vi "from string.vi"(8 "error in":errorcluster, 9 "data":string, 10 "version":string, 11 "Special Test configuration":refnum<class "Special Test configuration.lvclass">) -> (0 "error out":errorcluster, 3 "Special Test configuration out":refnum<class "Special Test configuration.lvclass">)   [LabVIEW 2025, in "Special Test.lvlib" / "Special Test configuration.lvclass"]
doc: "Provides an interface for loading a module configuration from a file or other serialized data source. It is recommended that all children of this class store data in two sets--data required for its own initialization, and any data required for parent initialization--and that each implementation uses the <b>Call Parent Method</b> primitive to de-serialize parent information.Copyright 2017 National Instruments Corporation\n\nLicensed under the Apache License, Version 2.0 (the \"License\"); you may not use this file except in compliance with the License. You may obtain a copy of the License at http://www.apache.org/licenses/LICENSE-2.0\nUnless required by applicable law or agreed to in writing, software distributed under the License is distributed on an \"AS IS\" BASIS, WITHOUT WARRANTIES OR CONDITIONS OF ANY KIND, either express or implied. See the License for the specific language governing permissions and limitations under the License."
uses:
  Special Test configuration.lvclass
  Test Info.ctl
  Special Test configuration.lvclass/Special Test configuration.ctl
  Users/Public/Documents/Sandia National Labs/TSS Plugin/CEF.lvlibp/serializable configuration/CEF_serializable configuration.lvclass
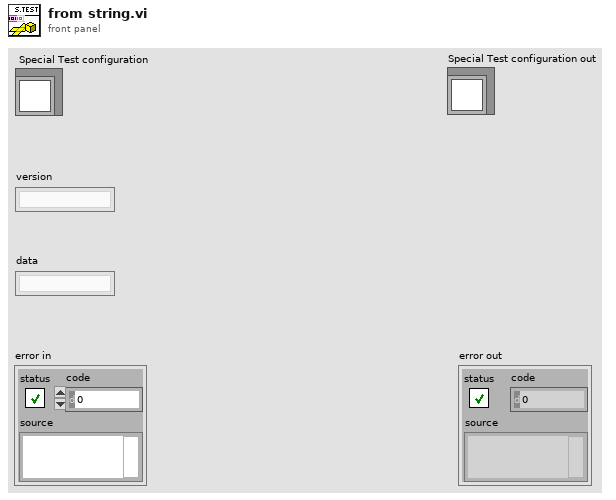
[diagram p1: front panel]
types:
  T1 = typedef "Special Test.lvlib/Special Test configuration.lvclass/Test Info.ctl" = cluster{"General":cluster{"Location":string, "Operator":string}, "Doc":cluster{"Shorthand Test Name":string, "MRS Code":string, "P6 Test Activity Name":string, "Test Plan":string, "Wiring Diagram":string}, "Test Setup":cluster{"Series":string, "Test Code":string, "Test Group":string, "Config Type":string}, "Run":cluster{"Temperature":string, "Voltage":string, "Attempt":u32, "Test Run":string, "Pre-Test Notes":string, "Source Code":string, "During Environment":string, "Enable Dropouts":bool}}
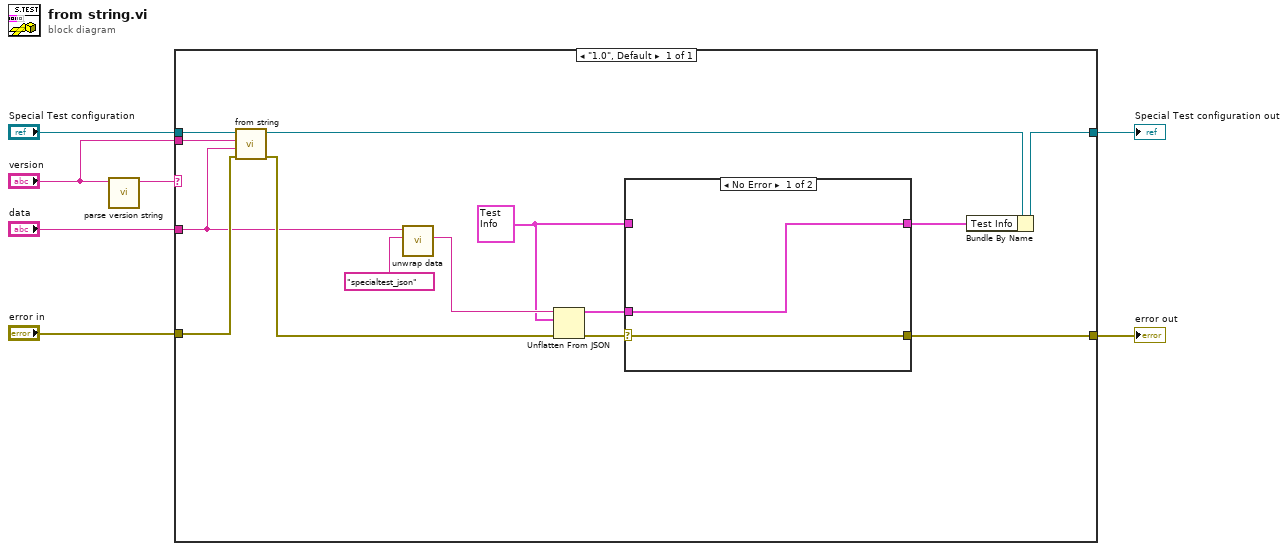
[diagram p0: block diagram]
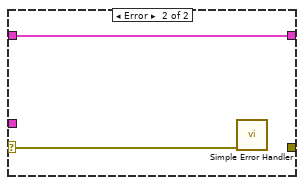
[diagram p2: hidden frame]
diagram:
  n1 = call "parse version string.vi"("full version"="version") -> ("major.minor version"=w3:string)  [unwired: 7 in, 3 out]
  n2 = case shown="\"1.0\", Default" w3 {
    tunnel: "Special Test configuration" -> [w21]
    tunnel: [w15] -> w4
    tunnel: "data" -> [w13]
    tunnel: "error in" -> [w19]
    tunnel: "version" -> [w14]
    tunnel: [w9] -> w1
    frame "1.0", Default {
      w8 = T1 {"General"={"Location"="840/176", "Operator"="JLee"}, "Doc"={"Shorthand Test Name"="RVIT1", "MRS Code"="EI020", "P6 Test Activity Name"="JST87NE_RVIT1", "Test Plan"="Added the Version section.", "Wiring Diagram"="HW Configuration"}, "Test Setup"={"Series"="N/A", "Test Code"="N/A", "Test Group"="SNL/NM", "Config Type"="Jung.L"}, "Run"={"Temperature"="Ambient", "Voltage"="Norminal", "Attempt"=1, "Test Run"="3AxxxxxA", "Pre-Test Notes"="TK3AxxxxA", "Source Code"="900", "During Environment"="1", "Enable Dropouts"=FALSE}} ("Test Info")
      n3 = call-parent "from string.vi"("error in"=w19, "data"=w13, "version"=w14, "CEF_Configuration in"=w21) -> ("error out"=w17:errorcluster, "CEF_Configuration out"=w16:refnum<class "Special Test configuration.lvclass">)  [unwired: 6 in]
      n4 = call "unwrap data.vi"("identifier"="specialtest_json" ("additional identifier"), "data to unwrap"=w13) -> ("unwrapped data"=w18:string)  [unwired: 8 in, 1 out]
      n5 = Unflatten From JSON(JSON string=w18, type and defaults=w8, error in (no error)=w17) -> (value=w11:T1, error out=w12:errorcluster)  [unwired: 4 in]
      n6 = case shown="No Error" w12 {
        selector: w12 -> [w22 w24]
        tunnel: w11 -> [w23 _]
        tunnel: [w23 w25] -> w10
        tunnel: w8 -> [_ w25]
        tunnel: [w22 _] -> w9
        frame No Error {
        }
        frame Error {
          n7 = call <vilib>:"Simple Error Handler.vi"("error in (no error)"=w24) -> ()  [unwired: 4 in, 5 out]
        }
      }
      n8 = Bundle By Name(cluster=w16, "Test Info"=w10) -> (w15:refnum<class "Special Test configuration.lvclass">)
    }
  }
  "error out" <- w1
  "Special Test configuration out" <- w4
